vi "Stop Neopixel FIFO.vi"(8 "Error In":errorcluster, 11 "Draw Frame In":refnum<class "Draw Frame.lvclass">) -> (0 "Error Out":errorcluster, 3 "Draw Frame Out":refnum<class "Draw Frame.lvclass">)   [LabVIEW 2019, in "Draw Frame.lvclass"]
uses:
  Draw Frame.lvclass
  Accessors/FPGA Reference/Get FPGA Reference.vi
  <vilib>/Utility/error.llb/Error Cluster From Error Code.vi
  Public/Controls/FPGA Reference.ctl
  <vilib>/rvi/interface/nirviMethod/nirviMethod.xnode
  <vilib>/FPGAPlugInAG/Dynamic/niLvFpga_StopFifo_Dynamic.vi
  <vilib>/rvi/errors/niLvFpgaMergeErrorWithErrorCode.vi
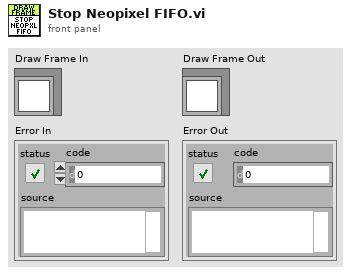
[diagram p1: front panel]
types:
  T1 = typedef "Draw Frame.lvclass/FPGA Reference.ctl" = refnum<k20>
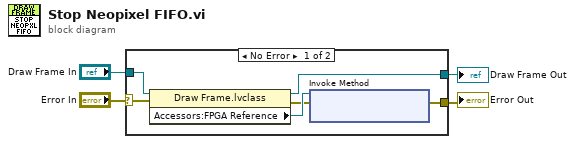
[diagram p0: block diagram]
diagram:
  n1 = case shown="No Error" "Error In" {
    selector: "Error In" -> [w8 w11]
    tunnel: [w5 w11] -> w4
    tunnel: [w10 w12] -> w3
    tunnel: "Draw Frame In" -> [w9 w12]
    frame No Error {
      n2 = property class="Draw Frame.lvclass"(reference=w9, error in=w8) -> (reference out=w10:refnum<class "Draw Frame.lvclass">, error out=w6:errorcluster, "Accessors:FPGA Reference"=w7:T1)
      n3 = xnode "Invoke Method"("FPGA VI Reference In"=w7, "error in"=w6) -> ("error out"=w5:errorcluster)  [unwired: 1 out]
    }
    frame Error {
    }
  }
  "Error Out" <- w4
  "Draw Frame Out" <- w3
